vi "Cam DeInit Done.vi"(8 "error in (no error)":errorcluster, 10 "InstrumentData":T1={"Exposure"=0.0, "Gain"=0.0, "Image XDim"=0, "Image YDim"=0, "Pixel Size"=0.0, "Image Type"=7} {"Image Type" items=["Grayscale (U8)", "Grayscale (U16)"]}, 11 "Camera_Controller in":refnum<class "Camera_Controller.lvclass">) -> (0 "error out":errorcluster, 3 "Camera_Controller out":refnum<class "Camera_Controller.lvclass">)   [LabVIEW 2023, in "CameraLibrary.lvlib" / "Camera_Controller.lvlib" / "Camera_Controller.lvclass"]
uses:
  Camera_Controller.lvclass
  typedefs/Camera_Init_Params.ctl
  typedefs/typedefs.lvlib
  typedefs/Image Type.ctl
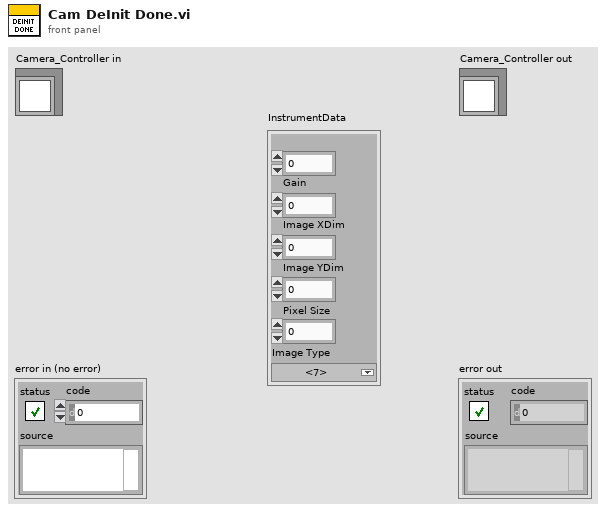
[diagram p1: front panel]
types:
  T1 = typedef "typedefs.lvlib/Camera_Init_Params.ctl" = cluster{"Exposure":dbl, "Gain":dbl, "Image XDim":u16, "Image YDim":u16, "Pixel Size":sgl, "Image Type":T2}
  T2 = typedef "typedefs.lvlib/Image Type.ctl" = u32
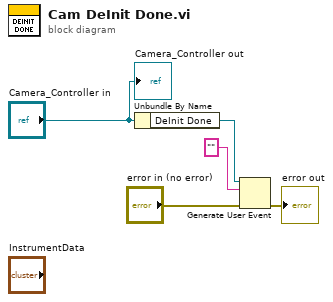
[diagram p0: block diagram]
diagram:
  n1 = Unbundle By Name("Camera_Controller in") -> ("DeInit Done"=w2:refnum<user-event>)
  n2 = Generate User Event(user event=w2, event data cluster="" ("event data"), error in="error in (no error)") -> (error out=→"error out":errorcluster)  [unwired: 1 in, 1 out]
  "Camera_Controller out" <- "Camera_Controller in"
